vi "Send Remote Transmission Request.vi"(8 "error in":errorcluster, 10 "Node ID":u8, 11 "Node Guard in":refnum<class "Node Guard.lvclass">) -> (0 "error out":errorcluster)   [LabVIEW 2020, in "CANopen.lvlib" / "Network Management.lvlib" / "Node Guard.lvlib" / "Node Guard.lvclass"]
uses:
  Node Guard.lvclass
  Node Guard.lvclass/Node Guard.ctl
  CANopen Message/CANopen Message.lvclass
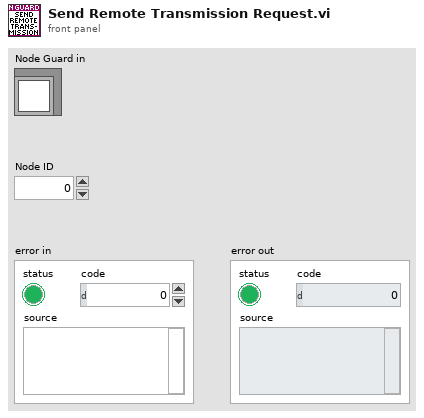
[diagram p1: front panel]
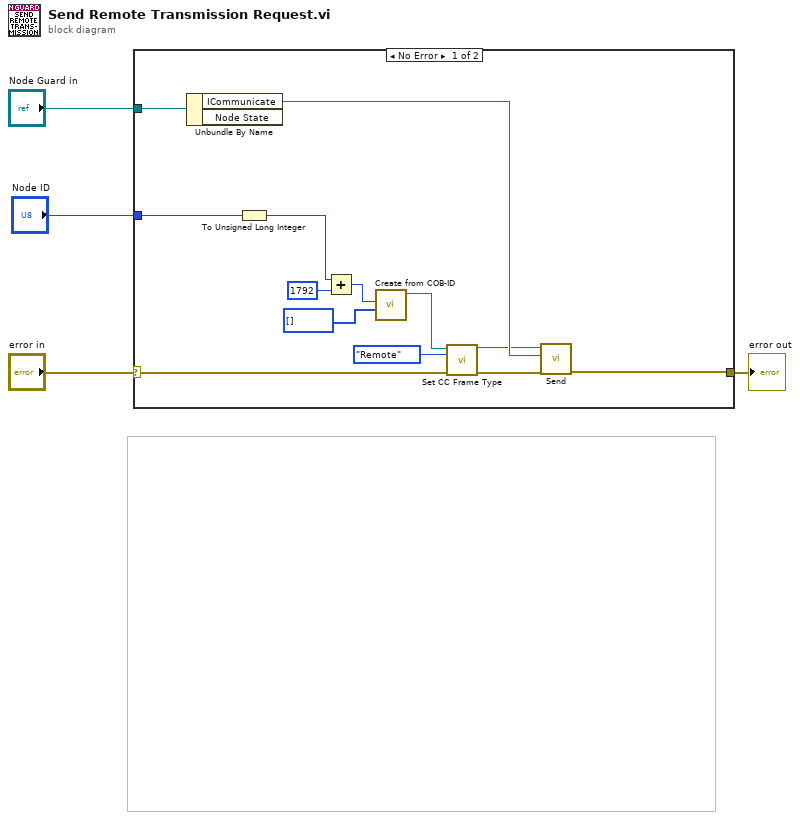
[diagram p0: block diagram]
diagram:
  n1 = case shown="No Error" "error in" {
    selector: "error in" -> [w8 w18]
    tunnel: [w15 w18] -> w2
    tunnel: "Node Guard in" -> [w17 _]
    tunnel: "Node ID" -> [w12 _]
    frame No Error {
      n2 = Unbundle By Name(w17) -> ("ICommunicate"=w16:refnum<class "ICommunicate.lvclass">)  [unwired: 1 out]
      n3 = To Unsigned Long Integer(number=w12) -> (unsigned 32bit integer=w11:u32)
      n4 = Add(x=w11, y=u32 1792 ("COB-ID")) -> (x+y=w13:u32)
      n5 = call "Create from COB-ID.vi"("Data"=u8[] [], "COB-ID"=w13) -> ("CANopen Message out"=w10:refnum<class "CANopen Message.lvclass">)  [unwired: 9 in]
      n6 = call "Set CC Frame Type.vi"("error in"=w8, "CC Frame Type"=enum8{"Data", "Remote", "Error", "Overload"}."Remote", "CANopen Message in"=w10) -> ("error out"=w9:errorcluster, "CANopen Message out"=w6:refnum<class "CANopen Message.lvclass">)  [unwired: 7 in]
      n7 = call "Send.vi"("error in"=w9, "ICommunicate"=w16, "CANopen Message in"=w6) -> ("error out"=w15:errorcluster)  [unwired: 7 in, 1 out]
    }
    frame Error {
    }
  }
  "error out" <- w2
